vi "check can.vi"(11 "Output Array":string[][](array[string])) -> (1 "Numeric":u16, 2 "element":string, 3 "element 2":string, 4 "output 3":u16, 5 "output 5":u16, 6 "output 4":u16)   [LabVIEW 2014]
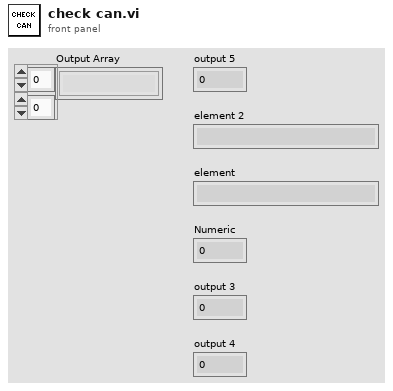
[diagram p1: front panel]
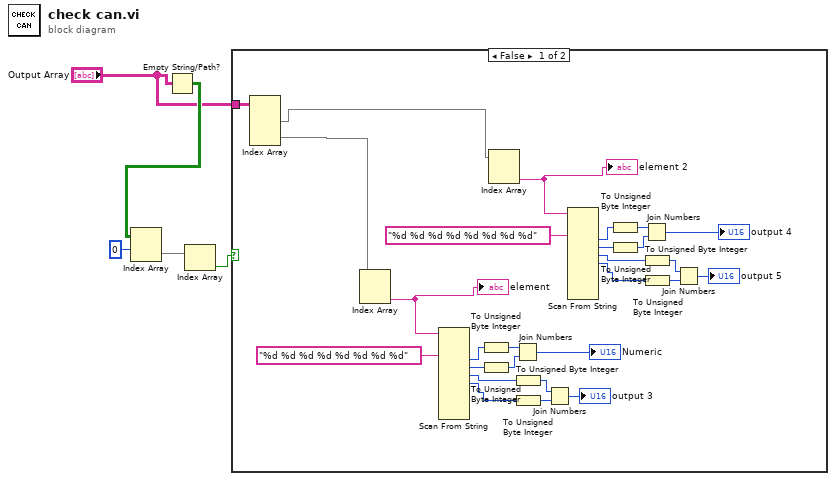
[diagram p0: block diagram]
diagram:
  n1 = Empty String/Path?(string/path="Output Array") -> (empty?=w5:bool[][])
  n2 = Index Array(array=w5, index (row)=0) -> (element=w3:bool[])  [unwired: 1 in]
  n3 = Index Array(array=w3) -> (element=w2:bool)  [unwired: 1 in]
  n4 = case shown="False" w2 {
    tunnel: "Output Array" -> [w6 _]
    frame False {
      n5 = Index Array(array=w6) -> (element #1=w7:string[], element #2=w8:string[])  [unwired: 4 in]
      n6 = Index Array(array=w8) -> (element #2=w10:string)  [unwired: 2 in, 1 out]
      "element" <- w10
      n7 = Scan From String(format string="%d %d %d %d %d %d %d %d", input string=w10) -> (output 1=w16:i32, output 2=w17:i32, output 3=w18:i32, output 4=w19:i32)  [unwired: 14 in, 3 out]
      n8 = To Unsigned Byte Integer(number=w16) -> (unsigned 8bit integer=w14:u8)
      n9 = To Unsigned Byte Integer(number=w17) -> (unsigned 8bit integer=w13:u8)
      n10 = Index Array(array=w7) -> (element #2=w22:string)  [unwired: 2 in, 1 out]
      "element 2" <- w22
      n11 = Join Numbers(hi=w14, lo=w13) -> ((hi.lo)=→"Numeric":u16)
      n12 = To Unsigned Byte Integer(number=w18) -> (unsigned 8bit integer=w12:u8)
      n13 = To Unsigned Byte Integer(number=w19) -> (unsigned 8bit integer=w11:u8)
      n14 = Join Numbers(hi=w12, lo=w11) -> ((hi.lo)=→"output 3":u16)
      n15 = Scan From String(format string="%d %d %d %d %d %d %d %d", input string=w22) -> (output 1=w28:i32, output 2=w29:i32, output 3=w30:i32, output 4=w31:i32)  [unwired: 14 in, 3 out]
      n16 = To Unsigned Byte Integer(number=w28) -> (unsigned 8bit integer=w26:u8)
      n17 = To Unsigned Byte Integer(number=w29) -> (unsigned 8bit integer=w25:u8)
      n18 = Join Numbers(hi=w26, lo=w25) -> ((hi.lo)=→"output 4":u16)
      n19 = To Unsigned Byte Integer(number=w30) -> (unsigned 8bit integer=w24:u8)
      n20 = To Unsigned Byte Integer(number=w31) -> (unsigned 8bit integer=w23:u8)
      n21 = Join Numbers(hi=w24, lo=w23) -> ((hi.lo)=→"output 5":u16)
    }
    frame True {
    }
  }
